vi "is_specific_error.vi"(2 "Boolean":bool, 3 "error in (no error)":errorcluster) -> (7 "error out":errorcluster)   [LabVIEW 2018]
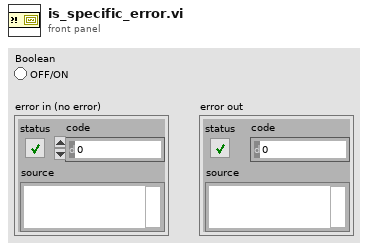
[diagram p1: front panel]
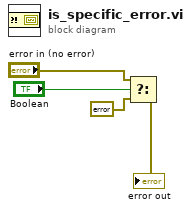
[diagram p0: block diagram]
diagram:
  n1 = Select(t="error in (no error)", s="Boolean", f=errorcluster {"status"=FALSE, "code"=0, "source"=""} ("error out")) -> (s? t:f=→"error out":errorcluster)
